vi "Fetch (SGL Array).vi"(6 "default timestamp":timestamp, 7 "PV name":string, 8 "error in":errorcluster, 10 "default value":sgl[](array[numeric]), 11 "Server in":refnum<class "Server.lvclass">) -> (0 "error out":errorcluster, 2 "value":sgl[](array[numeric]), 3 "Server out":refnum<class "Server.lvclass">, 4 "timestamp":timestamp)   [LabVIEW 2020, in "PV Access.lvlib" / "PVA Server.lvlib" / "Server.lvclass"]
uses:
  Server.lvclass
  PV Data/PV Data/PV Data.lvclass
  Source/Source.lvclass
  e690ada3-32d5-4897-ad72-20d0005fb086.vi
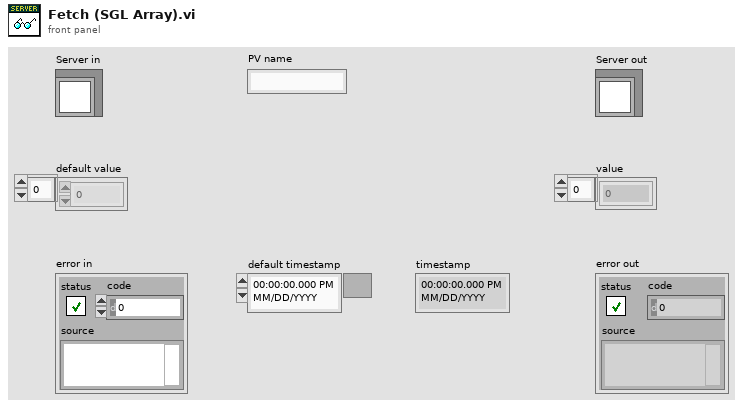
[diagram p1: front panel]
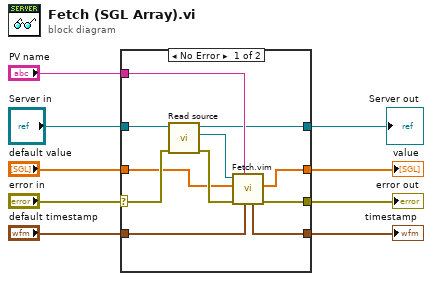
[diagram p0: block diagram]
diagram:
  n1 = case shown="No Error" "error in" {
    selector: "error in" -> [w18 w22]
    tunnel: [w20 w22] -> w9
    tunnel: "PV name" -> [w19 _]
    tunnel: [w17 w21] -> w6
    tunnel: "Server in" -> [w15 w24]
    tunnel: [w14 w24] -> w4
    tunnel: "default value" -> [w12 w23]
    tunnel: [w11 w23] -> w2
    tunnel: "default timestamp" -> [w10 w21]
    frame No Error {
      n2 = call "Read source.vi"("error in (no error)"=w18, "Server in"=w15) -> ("error out"=w16:errorcluster, "Source"=w13:refnum<class "Source.lvclass">, "Server out"=w14:refnum<class "Server.lvclass">)  [unwired: 7 in]
      n3 = call "Fetch.vim"("default timestamp"=w10, "PV name"=w19, "error in"=w16, "default"=w12, "Source in"=w13) -> ("error out"=w20:errorcluster, "value"=w11:sgl[], "timestamp"=w17:timestamp)  [unwired: 3 in, 1 out]
    }
    frame Error {
    }
  }
  "Server out" <- w4
  "error out" <- w9
  "timestamp" <- w6
  "value" <- w2
